vi "XY_string_generator.vi"() -> ()   [LabVIEW 2020]
uses:
  typedefs/typedef_XY_tiling.ctl
  pan-ASLM project/type_defs/Laser_toggles_typedef.ctl
  Global stop DAQ.vi
panel:
  out "String":string
  out "error OUT":errorcluster
  out "string array":string[](array[string])
  out "number":dbl
  out "substring":string
  in  "Laser Toggles":T1={"Laser 488 nm power"=0.0, "Laser 560 nm power"=0.0, "Laser 595 nm power"=0.0, "Laser 642 nm power"=0.0, "Laser 560 order selection"=2, "Laser 595 order selection"=0, "Laser 642 order selection"=0, "Laser 488 order selection"=1} {"Laser 488 order selection" items=["Not active", "1", "2", "3", "4"]; "Laser 642 order selection" items=["Not active", "1", "2", "3", "4"]; "Laser 595 order selection" items=["Not active", "1", "2", "3", "4"]; "Laser 560 order selection" items=["Not active", "1", "2", "3", "4"]; "Laser 642 nm power" min=0.0 max=5.0 scale=0.0..100.0; "Laser 595 nm power" min=0.0 max=5.0 scale=0.0..100.0; "Laser 560 nm power" min=0.0 max=5.0 scale=0.0..100.0; "Laser 488 nm power" min=0.0 max=5.0 scale=0.0..100.0}
  out "Numeric":i32
  in  "stop":bool
  out "element":string
  out "size(s)":i32
  in  "XY acquisition":T2={"Number of tiles in X"=3.0, "Number of tiles in Y"=3.0, "Step size XY (µm)"=500.0, "Acquire XY-tiling"=FALSE, "Moving time (ms)"=1000.0}
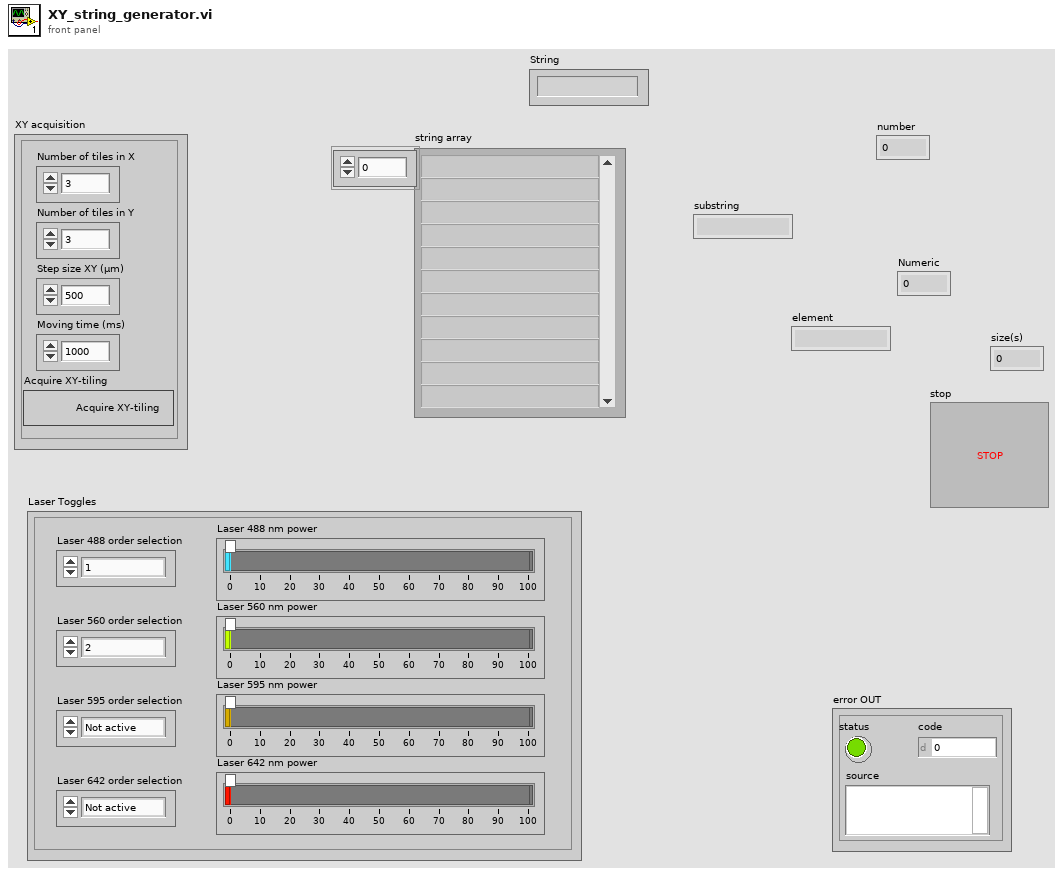
[diagram p1: front panel]
types:
  T1 = typedef "Laser_toggles_typedef.ctl" = cluster{"Laser 488 nm power":dbl, "Laser 560 nm power":dbl, "Laser 595 nm power":dbl, "Laser 642 nm power":dbl, "Laser 560 order selection":u16, "Laser 595 order selection":u16, "Laser 642 order selection":u16, "Laser 488 order selection":u16}
  T2 = typedef "typedef_XY_tiling.ctl" = cluster{"Number of tiles in X":dbl, "Number of tiles in Y":dbl, "Step size XY (µm)":dbl, "Acquire XY-tiling":bool, "Moving time (ms)":dbl}
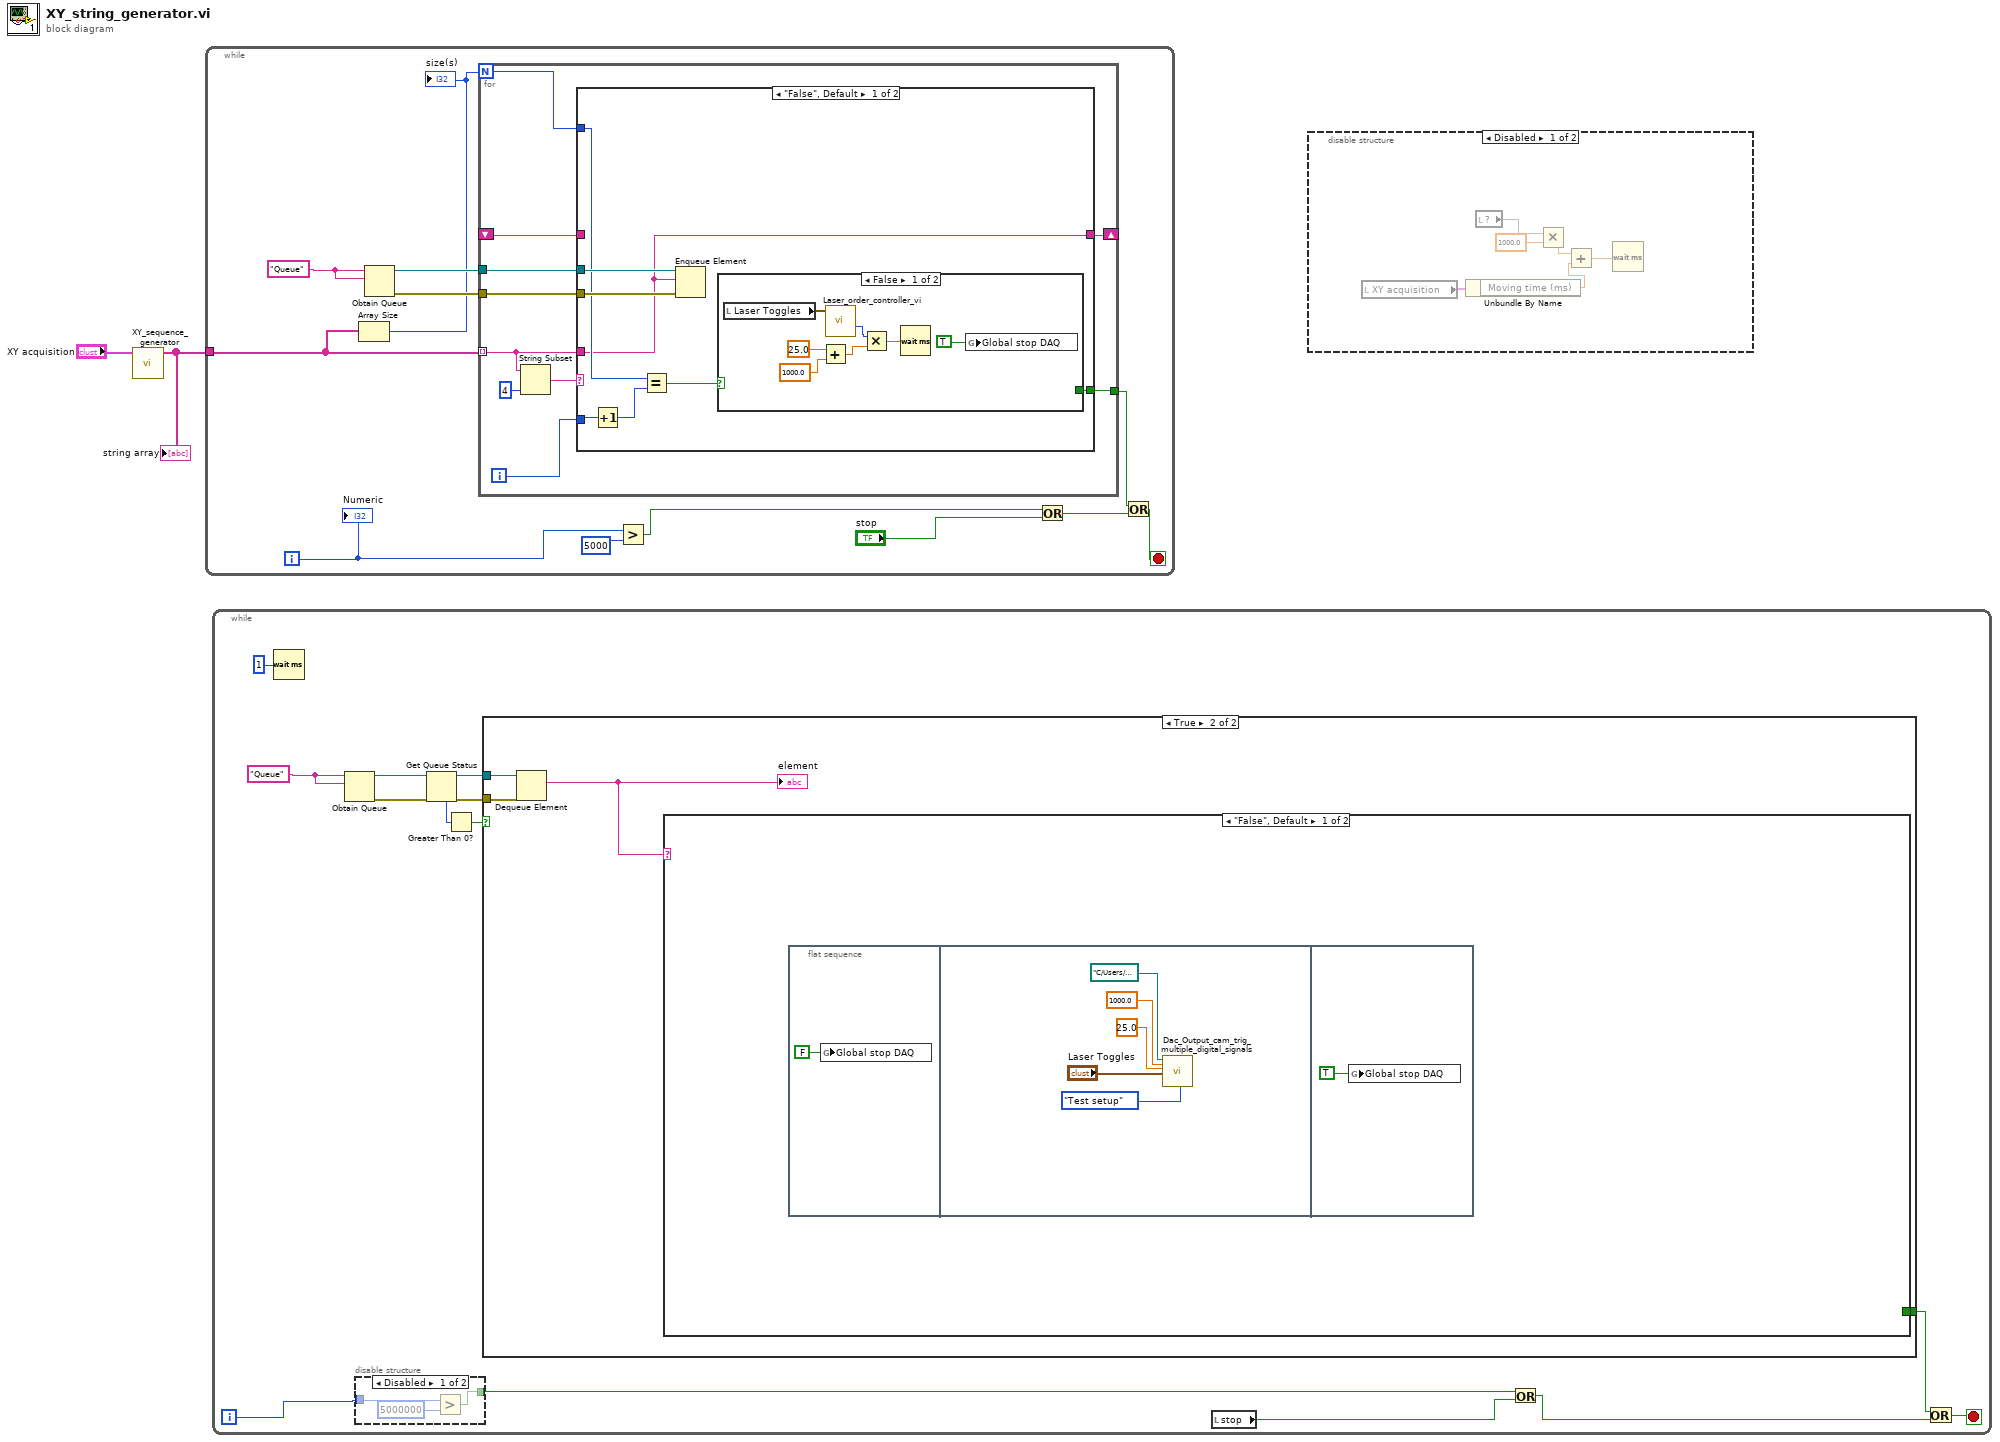
[diagram p0: block diagram]
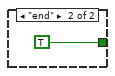
[diagram p5: hidden frame]
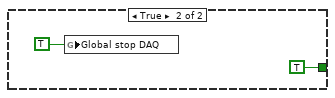
[diagram p6: hidden frame]
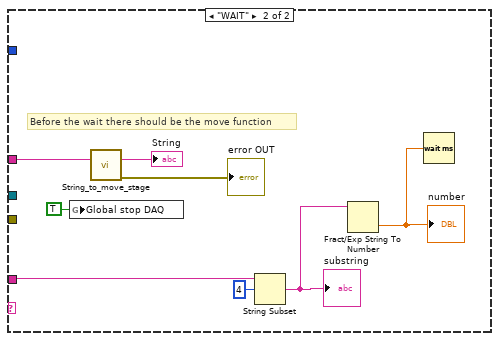
[diagram p7: hidden frame]
diagram:
  n1 = call "XY_sequence_generator.vi"("XY acquisition"="XY acquisition") -> ("string array"=w2:string[])  [unwired: 10 in]
  "string array" <- w2
  n2 = while {
    tunnel: w2 -> [w13]
    i -> [w4]
    stop <- w10 stop-if-true
    w14 = "Queue" ("name (unnamed)")
    n3 = Array Size(array=w13) -> (size(s)=w8:i32)
    "size(s)" <- w8
    n4 = Obtain Queue(name (unnamed)=w14, element data type=w14) -> (queue out=w12:refnum<queue>, error out=w11:errorcluster)  [unwired: 3 in, 1 out]
    n5 = for {
      N: w8 -> [w22]
      tunnel: w13 -> [w19] mode=indexing
      tunnel: w12 -> [w24]
      tunnel: w11 -> [w23]
      tunnel: [w21] -> w9
      shift-right: [w16] -> _
      shift-left: _ -> [w15]
      i -> [w20]
      n6 = String Subset(string=w19, length (rest)=4 ("length (rest)")) -> (substring=w18:string)  [unwired: 1 in]
      n7 = case shown="\"False\", Default" w18 {
        tunnel: w24 -> [w32 _]
        tunnel: w23 -> [w31 _]
        tunnel: w19 -> [w25 w49]
        tunnel: w22 -> [w30 _]
        tunnel: [w28 _] -> w21
        tunnel: w20 -> [w26 _]
        tunnel: [w25 _] -> w16
        tunnel: w15 -> [_ w44]
        frame "False", Default {
          n8 = Increment(x=w26) -> (x+1=w27:i32)
          n9 = Equal?(x=w30, y=w27) -> (x = y?=w29:bool)
          n10 = Enqueue Element(queue=w32, element=w25, error in (no error)=w31) -> ()  [unwired: 1 in, 3 out]
          n11 = case shown="False" w29 {
            tunnel: [_ TRUE] -> w28
            frame False {
              n12 = local read "Laser Toggles"() -> (w37:T1)
              n13 = Add(x=25.0, y=1000.0) -> (x+y=w35:dbl)
              n14 = call "Laser_order_controller_vi.vi"("Laser Toggles"=w37) -> ("Active lasers"=w36:i16)  [unwired: 8 in, 2 out]
              n15 = Multiply(x=w36, y=w35) -> (x*y=w39:dbl)
              n16 = Wait (ms)(milliseconds to wait=w39) -> ()  [unwired: 1 out]
              n17 = global write "Global stop DAQ.vi" "Global stop DAQ"(TRUE ("Global stop DAQ")) -> ()
            }
            frame True {
              n18 = global write "Global stop DAQ.vi" "Global stop DAQ"(TRUE ("Global stop DAQ")) -> ()
            }
          }
        }
        frame "WAIT" {
          # "Before the wait there should be the move function"
          n19 = global write "Global stop DAQ.vi" "Global stop DAQ"(TRUE ("Global stop DAQ")) -> ()
          n20 = call "String_to_move_stage.vi"("Movement string"=w44) -> ("String"=→"String":string, "error OUT"=→"error OUT":errorcluster)  [unwired: 12 in, 1 out]
          n21 = String Subset(string=w49, offset (0)=4) -> (substring=w47:string)  [unwired: 1 in]
          "substring" <- w47
          n22 = Fract/Exp String To Number(string=w47) -> (number=w45:dbl)  [unwired: 3 in, 1 out]
          "number" <- w45
          n23 = Wait (ms)(milliseconds to wait=w45) -> ()  [unwired: 1 out]
        }
      }
    }
    n24 = Greater?(x=w4, y=5000) -> (0:w3:bool)
    n25 = Or(x=w3, y="stop") -> (x .or. y?=w7:bool)
    n26 = Or(x=w9, y=w7) -> (x .or. y?=w10:bool)
    "Numeric" <- w4
  }
  n27 = while {
    i -> [w52]
    stop <- w55 stop-if-true
    w63 = "Queue" ("name (unnamed)")
    n28 = Wait (ms)(milliseconds to wait=u32 1) -> ()  [unwired: 1 out]
    n29 = Obtain Queue(name (unnamed)=w63, element data type=w63) -> (queue out=w62:refnum<queue>, error out=w61:errorcluster)  [unwired: 3 in, 1 out]
    n30 = disable-structure shown="Disabled" {
      disable-tunnel: w52 -> [w66 _]
      disable-tunnel: [w64 _] -> w51
      frame Disabled {
        n31 = Greater?(x=w66, y=5000000) -> (0:w64:bool)
      }
      frame Enabled {
      }
    }
    n32 = Get Queue Status(queue=w62, error in (no error)=w61) -> (queue out=w58:refnum<queue>, error out=w57:errorcluster, # elements in queue=w60:i32)  [unwired: 1 in, 5 out]
    n33 = Greater Than 0?(x=w60) -> (x > 0?=w59:bool)
    n34 = case shown="True" w59 {
      tunnel: w58 -> [_ w70]
      tunnel: w57 -> [_ w69]
      tunnel: [_ w67] -> w56
      frame False {
      }
      frame True {
        n35 = Dequeue Element(queue=w70, error in (no error)=w69) -> (element=w68:string)  [unwired: 1 in, 3 out]
        "element" <- w68
        n36 = case shown="\"False\", Default" w68 {
          tunnel: [_ TRUE] -> w67
          frame "False", Default {
            n37 = flat-sequence {
              frame #0 {
                n38 = global write "Global stop DAQ.vi" "Global stop DAQ"(FALSE ("Global stop DAQ")) -> ()
              }
              frame #1 {
                n39 = call "Dac_Output_cam_trig_multiple_digital_signals.vi"("File to read"=path "C:/Users/lpk27/Documents/pan-ASLMsynched/pan-ASLM/Calibration files/newcalibration_voice coil input_25msflyback.txt", "Image acquisition time (ms)"=1000.0, "Delay between frames"=25.0, "Laser Toggles"="Laser Toggles", "Setup"=enum16{"Test setup", "Microscope"}."Test setup") -> ()  [unwired: 14 in, 1 out]
              }
              frame #2 {
                n40 = global write "Global stop DAQ.vi" "Global stop DAQ"(TRUE ("Global stop DAQ")) -> ()
              }
            }
          }
          frame "end" {
          }
        }
      }
    }
    n41 = local read "stop"() -> (w53:bool)
    n42 = Or(x=w51, y=w53) -> (x .or. y?=w54:bool)
    n43 = Or(x=w56, y=w54) -> (x .or. y?=w55:bool)
  }
  n44 = disable-structure shown="Disabled" {
    frame Disabled {
      n45 = local read "XY acquisition"() -> (w80:T2)
      n46 = Unbundle By Name(w80) -> ("Moving time (ms)"=w81:dbl)
      n47 = local read item#-1() -> (w83)
      n48 = Multiply(x=w83, y=1000.0) -> (x*y=w84:dbl)
      n49 = Add(x=w84, y=w81) -> (x+y=w82:dbl)
      n50 = Wait (ms)(milliseconds to wait=w82) -> ()  [unwired: 1 out]
    }
    frame Enabled {
    }
  }
